vi "State wise behavior_MI.vi"(8 "error in (no error)":errorcluster, 9 "State":string, 10 "MIRecipeOpcodes":T1, 11 "VISA Refnum in":refnum<visa-resource-name>) -> (0 "error out":errorcluster, 3 "VISA Refnum out":refnum<visa-resource-name>)   [LabVIEW 2019, in "Machine Interface.lvclass"]
uses:
  Machine Interface.lvclass
  Controls/Machine Interface Config File Structure_MI.ctl
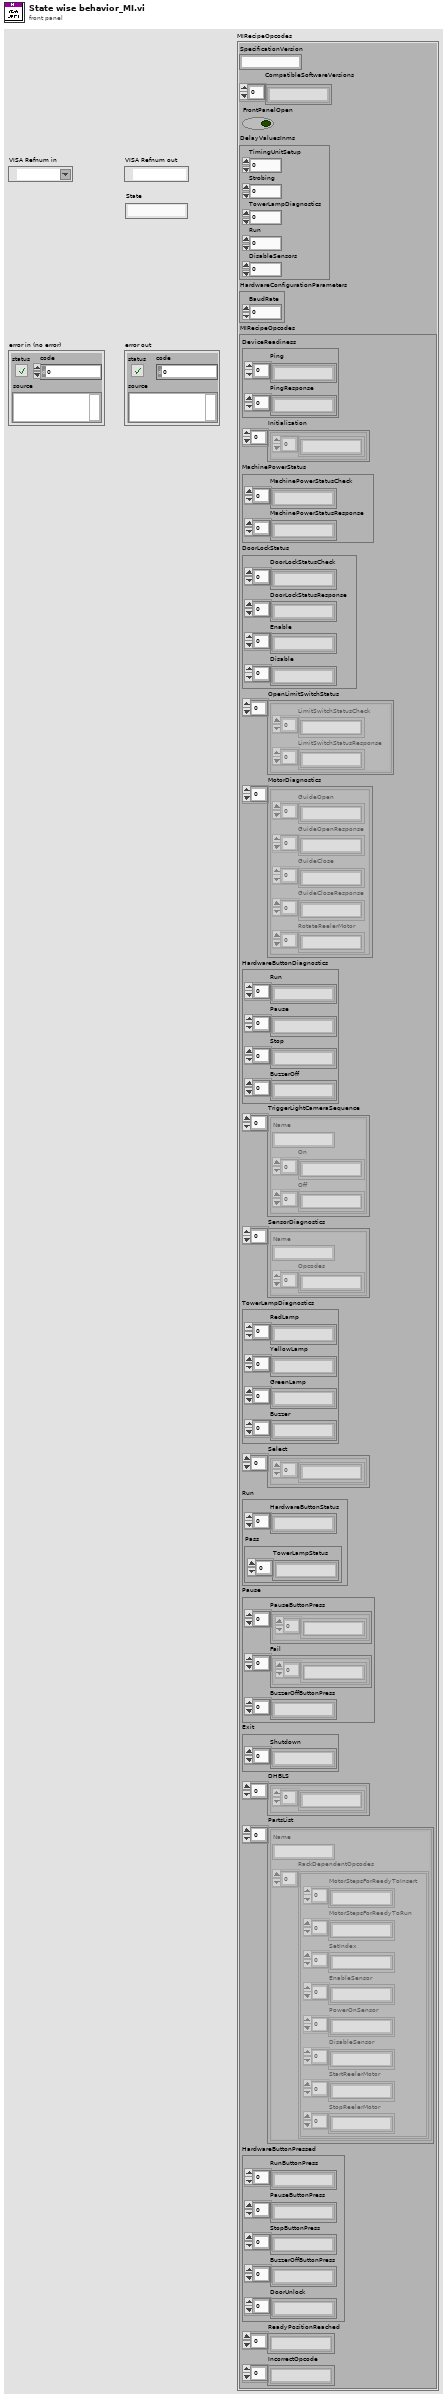
[diagram p1: front panel]
types:
  T1 = typedef "Machine Interface.lvclass/Machine Interface Config File Structure_MI.ctl" = cluster{"SpecificationVersion":string, "CompatibleSoftwareVersions":string[], "FrontPanelOpen":bool, "DelayValuesInms":cluster{"TimingUnitSetup":i32, "Strobing":i32, "TowerLampDiagnostics":i32, "Run":i32, "DisableSensors":i32}, "HardwareConfigurationParameters":cluster{"BaudRate":dbl}, "MIRecipeOpcodes":cluster{"DeviceReadiness":cluster{"Ping":string[], "PingResponse":string[]}, "Initialization":cluster{string[]}[], "MachinePowerStatus":cluster{"MachinePowerStatusCheck":string[], "MachinePowerStatusResponse":string[]}, "DoorLockStatus":cluster{"DoorLockStatusCheck":string[], "DoorLockStatusResponse":string[], "Enable":string[], "Disable":string[]}, "OpenLimitSwitchStatus":cluster{"LimitSwitchStatusCheck":string[], "LimitSwitchStatusResponse":string[]}[], "MotorDiagnostics":cluster{"GuideOpen":string[], "GuideOpenResponse":string[], "GuideClose":string[], "GuideCloseResponse":string[], "RotateReelerMotor":string[]}[], "HardwareButtonDiagnostics":cluster{"Run":string[], "Pause":string[], "Stop":string[], "BuzzerOff":string[]}, "TriggerLightCameraSequence":cluster{"Name":string, "On":string[], "Off":string[]}[], "SensorDiagnostics":cluster{"Name":string, "Opcodes":string[]}[], "TowerLampDiagnostics":cluster{"RedLamp":string[], "YellowLamp":string[], "GreenLamp":string[], "Buzzer":string[]}, "Select":cluster{string[]}[], "Run":cluster{"HardwareButtonStatus":string[], "Pass":cluster{"TowerLampStatus":string[]}}, "Pause":cluster{"PauseButtonPress":cluster{string[]}[], "Fail":cluster{string[]}[], "BuzzerOffButtonPress":string[]}, "Exit":cluster{"Shutdown":string[]}, "DHBLS":cluster{string[]}[], "PartsList":cluster{"Name":string, "RackDependentOpcodes":cluster{"MotorStepsForReadyToInsert":string[], "MotorStepsForReadyToRun":string[], "SetIndex":string[], "EnableSensor":string[], "PowerOnSensor":string[], "DisableSensor":string[], "StartReelerMotor":string[], "StopReelerMotor":string[]}[]}[], "HardwareButtonPressed":cluster{"RunButtonPress":string[], "PauseButtonPress":string[], "StopButtonPress":string[], "BuzzerOffButtonPress":string[], "DoorUnlock":string[]}, "ReadyPositionReached":string[], "IncorrectOpcode":string[]}}
  T2 = cluster{"RedLamp":string[], "YellowLamp":string[], "GreenLamp":string[], "Buzzer":string[]}
  T3 = cluster{"LimitSwitchStatusCheck":string[], "LimitSwitchStatusResponse":string[]}[]
  T4 = cluster{"LimitSwitchStatusCheck":string[], "LimitSwitchStatusResponse":string[]}
  T5 = cluster{"GuideOpen":string[], "GuideOpenResponse":string[], "GuideClose":string[], "GuideCloseResponse":string[], "RotateReelerMotor":string[]}[]
  T6 = cluster{"GuideOpen":string[], "GuideOpenResponse":string[], "GuideClose":string[], "GuideCloseResponse":string[], "RotateReelerMotor":string[]}
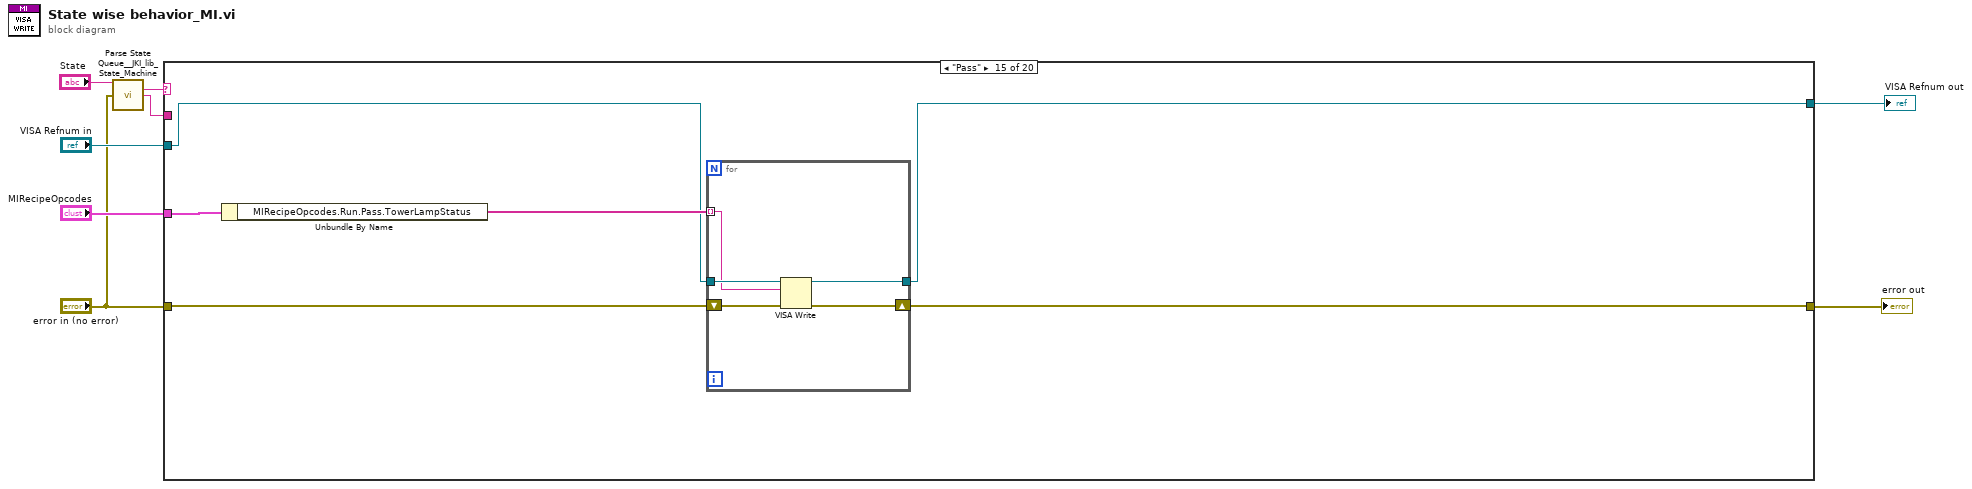
[diagram p0: block diagram]
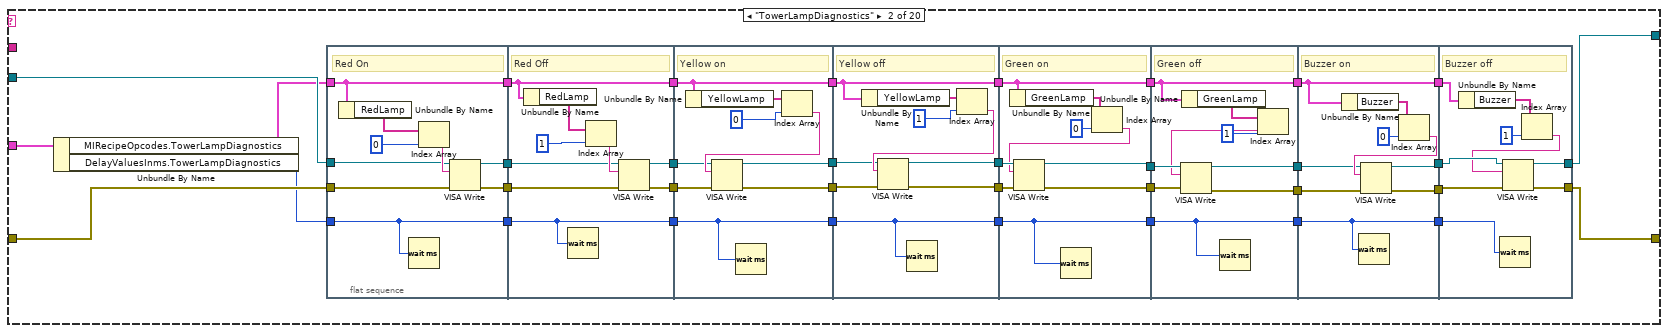
[diagram p3: hidden frame]
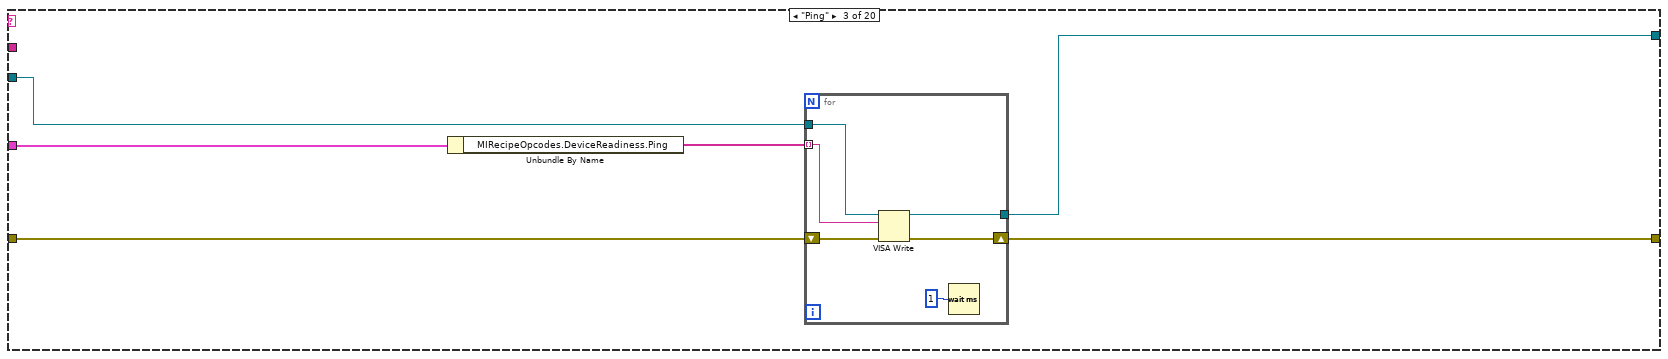
[diagram p4: hidden frame]
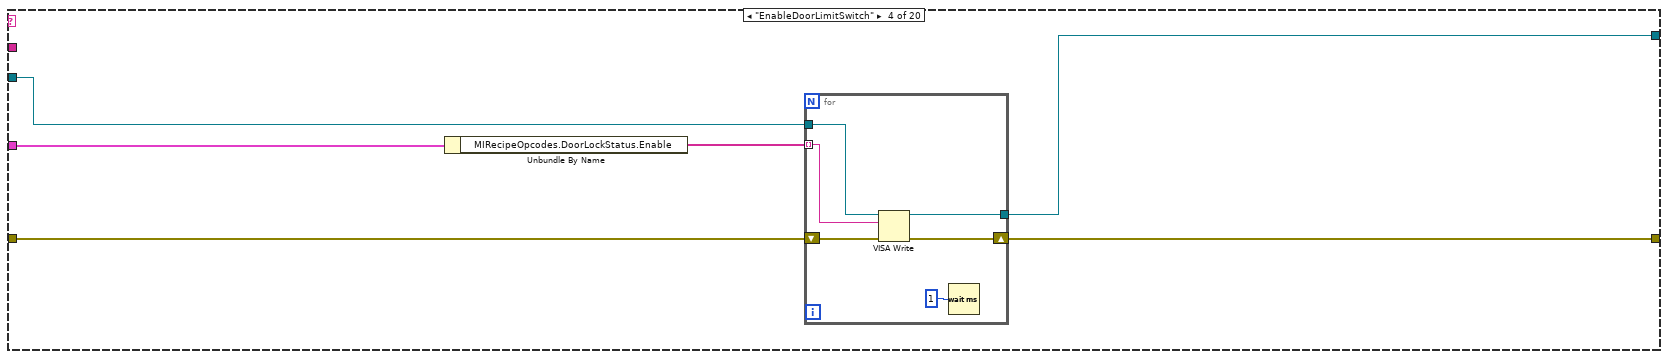
[diagram p5: hidden frame]
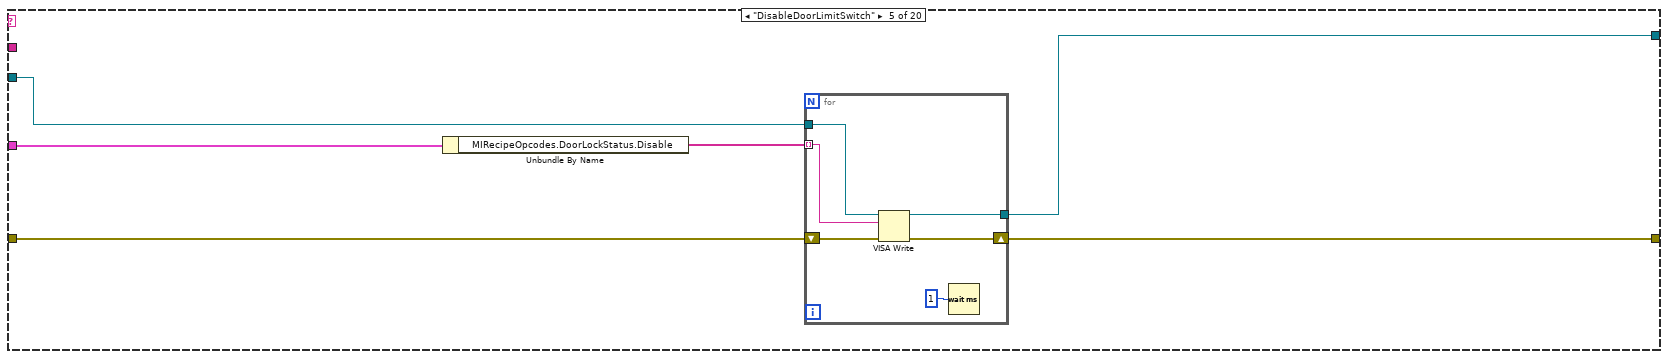
[diagram p6: hidden frame]
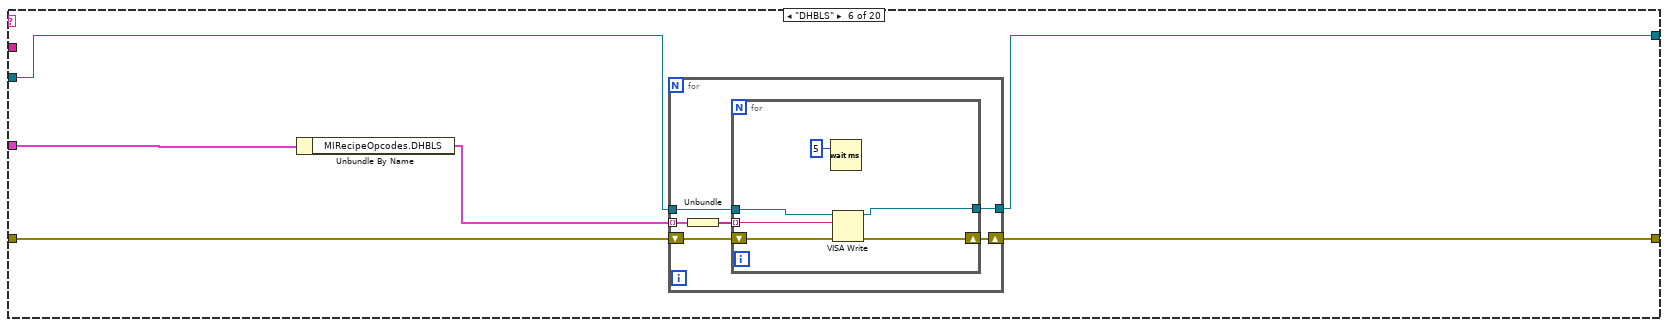
[diagram p7: hidden frame]
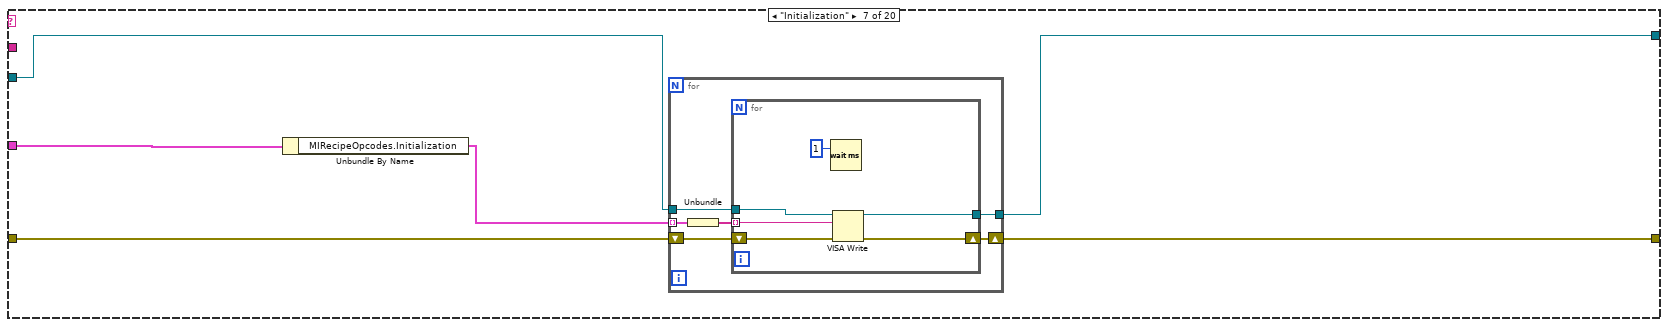
[diagram p8: hidden frame]
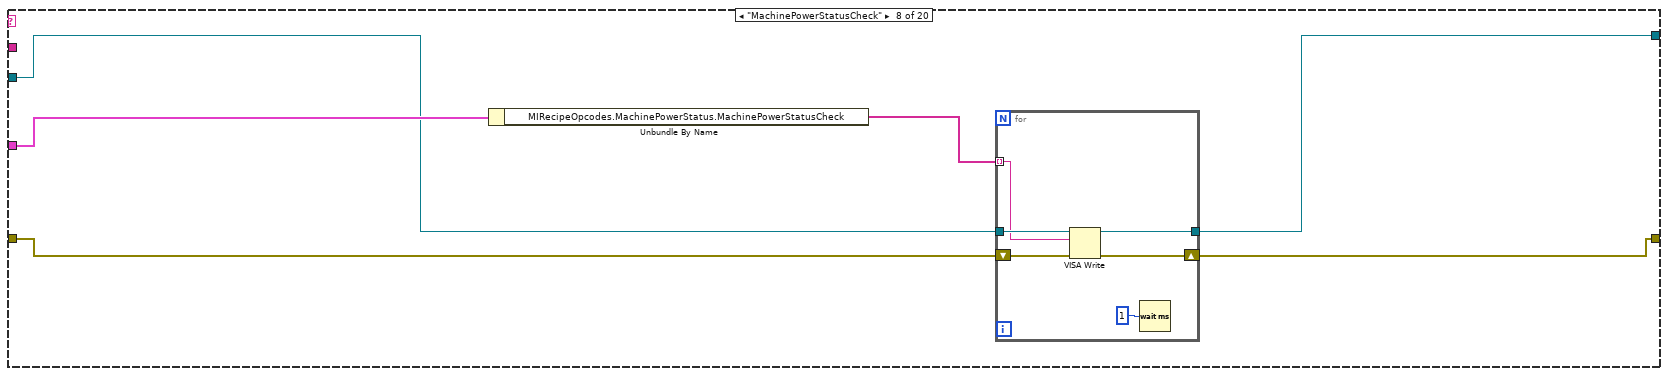
[diagram p9: hidden frame]
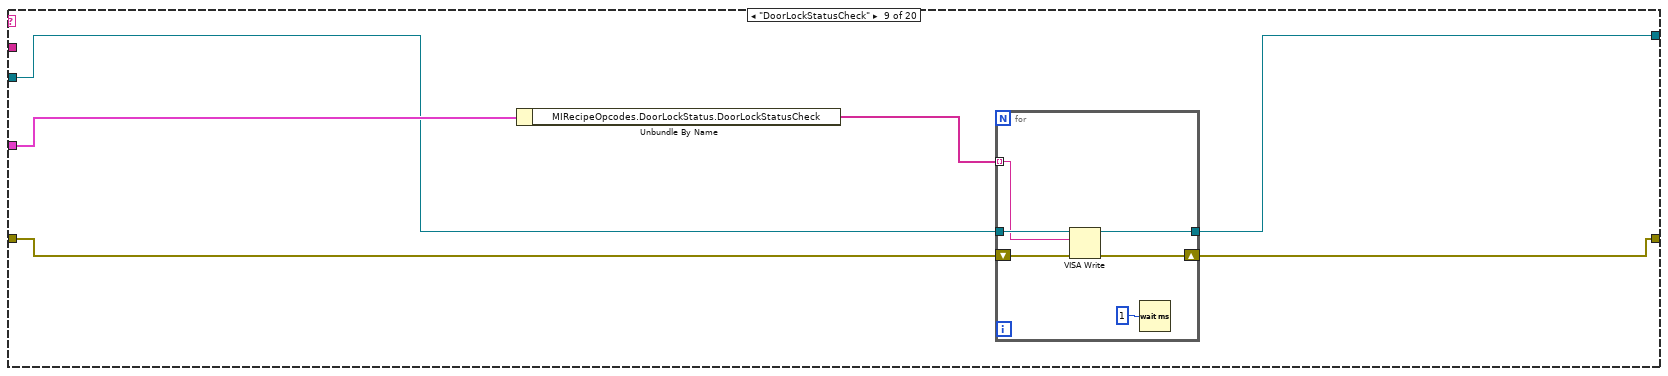
[diagram p10: hidden frame]
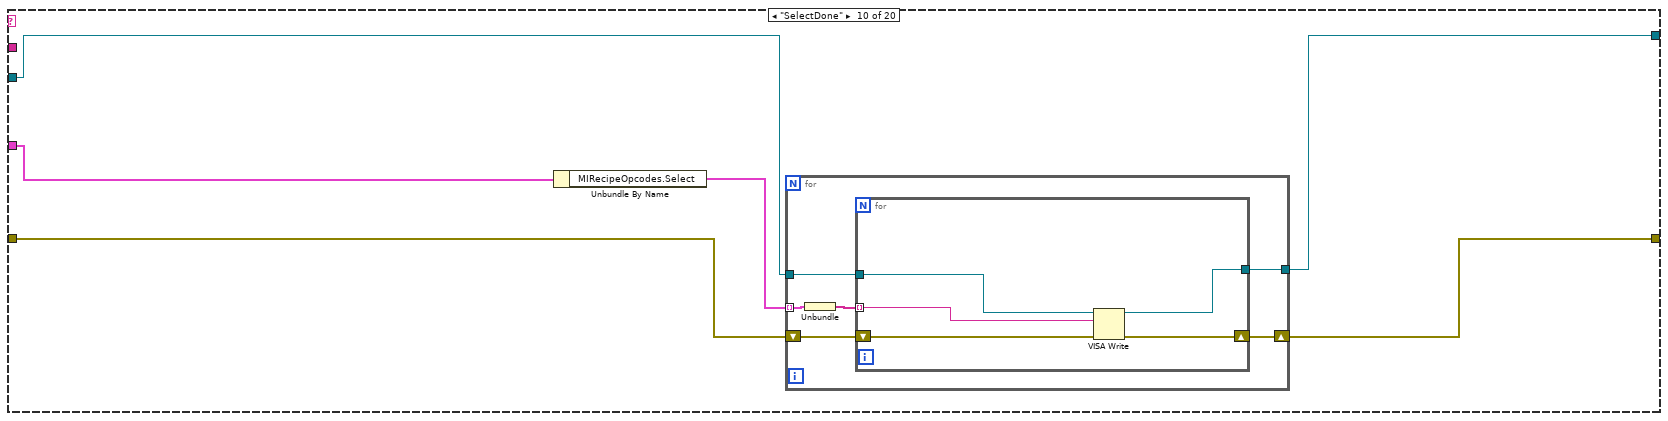
[diagram p11: hidden frame]
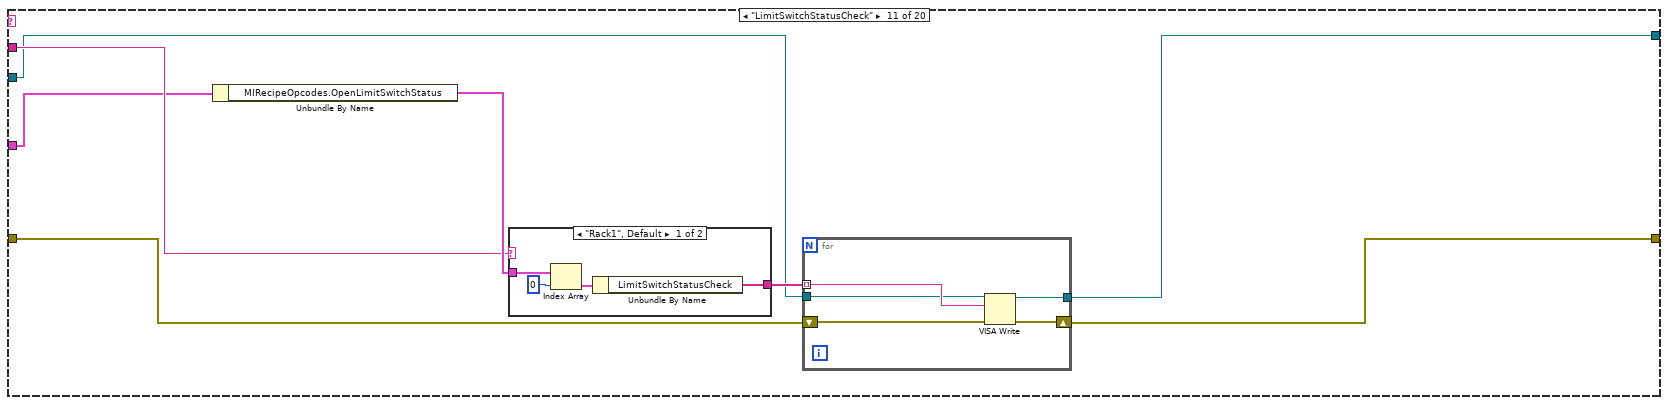
[diagram p12: hidden frame]
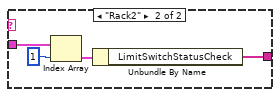
[diagram p13: hidden frame]
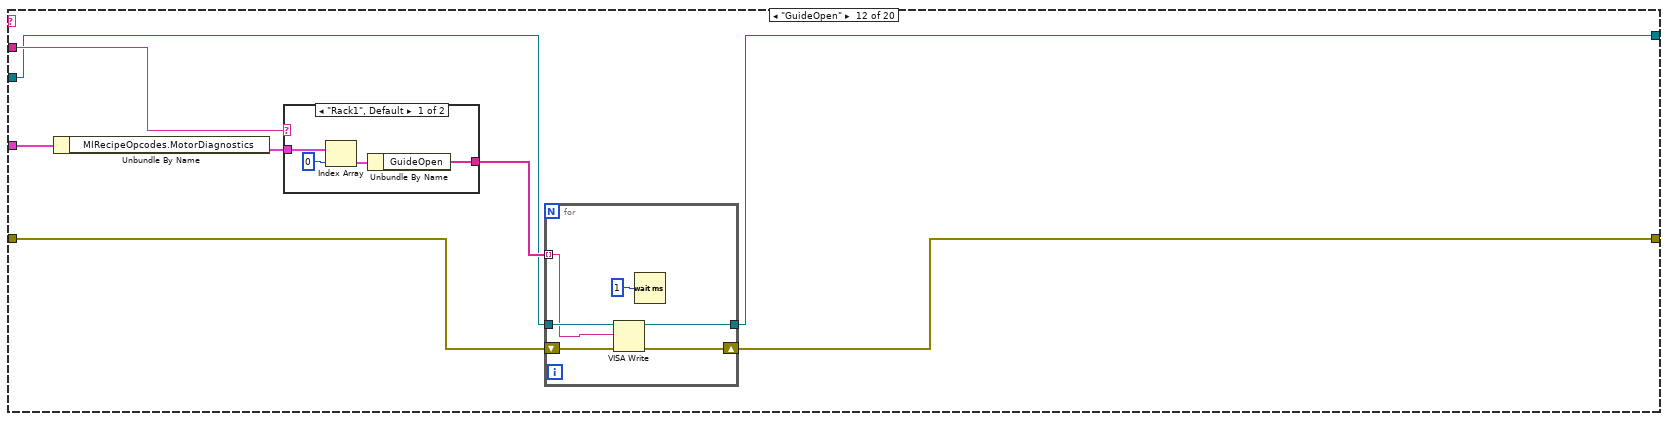
[diagram p14: hidden frame]
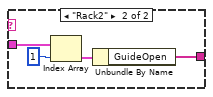
[diagram p15: hidden frame]
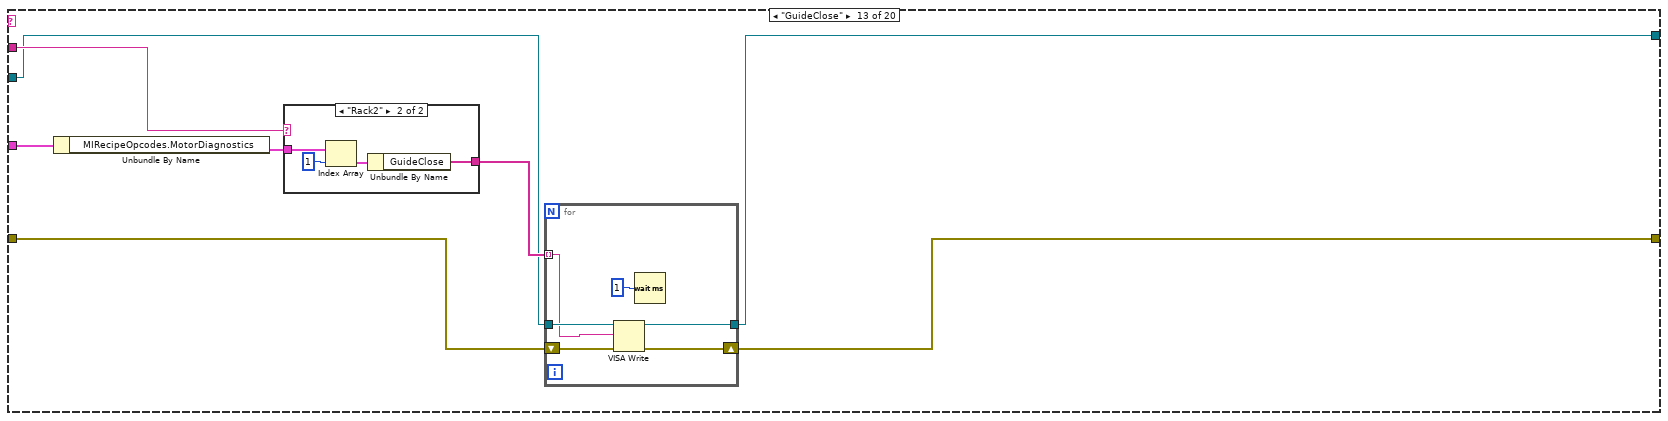
[diagram p16: hidden frame]
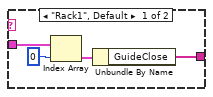
[diagram p17: hidden frame]
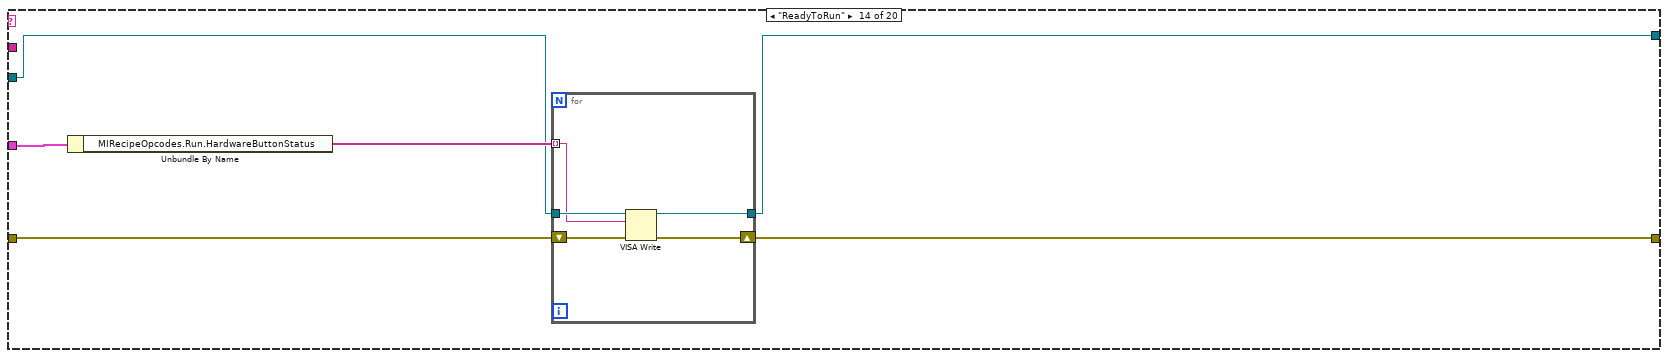
[diagram p18: hidden frame]
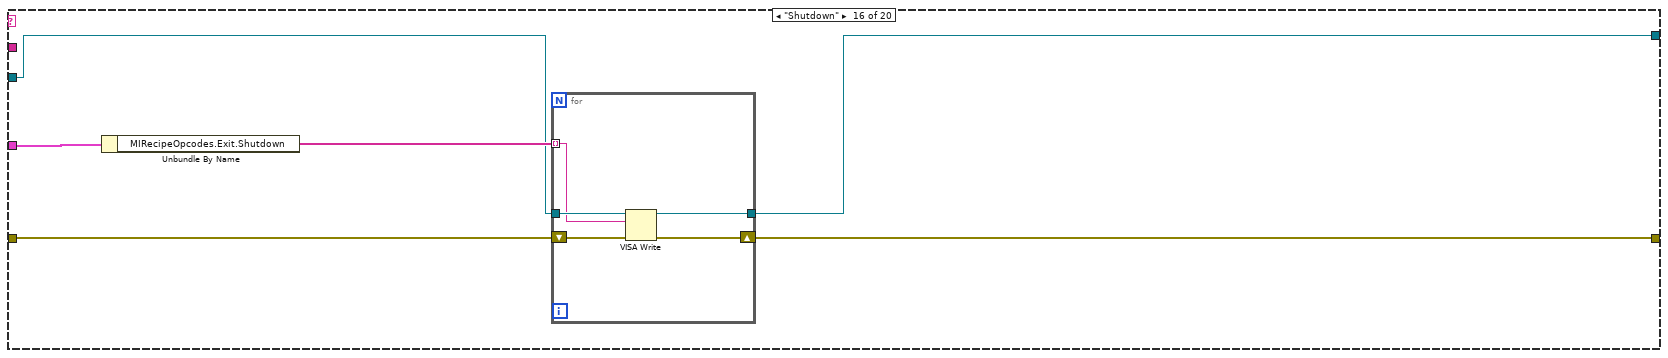
[diagram p19: hidden frame]
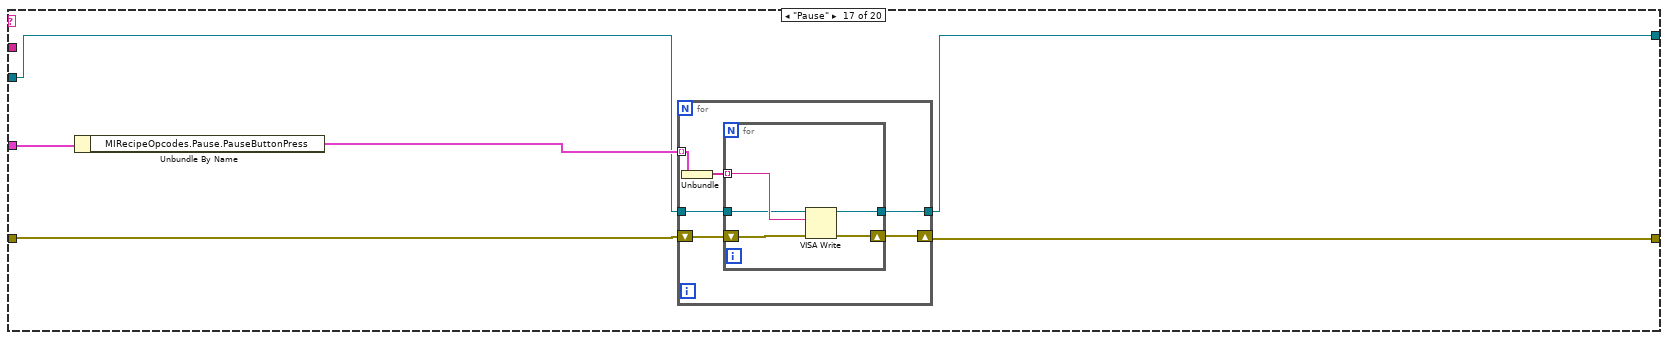
[diagram p20: hidden frame]
diagram:
  n1 = call <vilib>:"Parse State Queue__JKI_lib_State_Machine.vi"("State Queue"="State", "Error In (no error)"="error in (no error)") -> ("Current State"=w2:string, "Arguments"=w3:string)  [unwired: 11 in, 1 out]
  n2 = case shown="\"Pass\"" w2 {
    tunnel: "error in (no error)" -> [w10 w24 w121 w133 w145 w157 w175 w193 w205 w217 w234 w257 w279 w301 w312 w323 w332 w349 w368 w390]
    tunnel: [w9 w23 w118 w130 w142 w154 w172 w190 w202 w214 w231 w252 w274 w296 w307 w318 w329 w346 w363 w385] -> w8
    tunnel: [w10 w22 w120 w132 w144 w156 w174 w192 w204 w216 w233 w256 w278 w300 w311 w322 w331 w348 w367 w389] -> w1
    tunnel: "VISA Refnum in" -> [w9 w21 w119 w131 w143 w155 w173 w191 w203 w215 w232 w253 w275 w297 w308 w319 w330 w347 w364 w386]
    tunnel: "MIRecipeOpcodes" -> [_ w20 w122 w134 w146 w159 w177 w194 w206 w219 w235 w255 w277 w299 w310 w321 w334 w351 w366 w387]
    tunnel: w3 -> [_ _ _ _ _ _ _ _ _ _ w236 w258 w280 _ _ _ _ _ w369 _]
    frame Default {
    }
    frame "TowerLampDiagnostics" {
      n3 = Unbundle By Name(w20) -> ("MIRecipeOpcodes.TowerLampDiagnostics"=w19:T2, "DelayValuesInms.TowerLampDiagnostics"=w13:i32)
      n4 = flat-sequence {
        tunnel: w19 -> [w54]
        tunnel: [w54] -> w45
        tunnel: w24 -> [w51]
        tunnel: [w50] -> w44
        tunnel: w21 -> [w48]
        tunnel: [w47] -> w43
        tunnel: [w46] -> w14
        tunnel: w13 -> [w46]
        tunnel: [w58] -> w42
        tunnel: w45 -> [w58]
        tunnel: [w57] -> w41
        tunnel: w44 -> [w60]
        tunnel: w43 -> [w59]
        tunnel: [w56] -> w40
        tunnel: [w55] -> w15
        tunnel: w14 -> [w55]
        tunnel: [w69] -> w39
        tunnel: w42 -> [w69]
        tunnel: [w67] -> w38
        tunnel: w41 -> [w68]
        tunnel: w40 -> [w66]
        tunnel: [w65] -> w37
        tunnel: [w64] -> w16
        tunnel: w15 -> [w64]
        tunnel: [w78] -> w36
        tunnel: w39 -> [w78]
        tunnel: [w76] -> w35
        tunnel: w38 -> [w77]
        tunnel: w37 -> [w75]
        tunnel: [w74] -> w34
        tunnel: [w73] -> w17
        tunnel: w16 -> [w73]
        tunnel: [w90] -> w33
        tunnel: w36 -> [w90]
        tunnel: [w86] -> w32
        tunnel: w35 -> [w87]
        tunnel: w34 -> [w85]
        tunnel: [w83] -> w31
        tunnel: [w82] -> w18
        tunnel: w17 -> [w82]
        tunnel: [w99] -> w30
        tunnel: w33 -> [w99]
        tunnel: [w95] -> w29
        tunnel: w32 -> [w96]
        tunnel: w31 -> [w94]
        tunnel: [w92] -> w28
        tunnel: w18 -> [w91]
        tunnel: [w91] -> w11
        tunnel: [w108] -> w27
        tunnel: w30 -> [w108]
        tunnel: [w104] -> w26
        tunnel: w29 -> [w105]
        tunnel: w28 -> [w102]
        tunnel: [w101] -> w25
        tunnel: [w100] -> w12
        tunnel: w11 -> [w100]
        tunnel: w27 -> [w115]
        tunnel: w26 -> [w114]
        tunnel: [w113] -> w22
        tunnel: w25 -> [w112]
        tunnel: [w110] -> w23
        tunnel: w12 -> [w109]
        frame #0 {
          # "Red On"
          n5 = Unbundle By Name(w54) -> ("RedLamp"=w53:string[])
          n6 = Wait (ms)(milliseconds to wait=w46) -> ()  [unwired: 1 out]
          n7 = Index Array(array=w53, index=0) -> (element=w49:string)
          n8 = VISA Write(VISA resource name=w48, write buffer=w49, error in (no error)=w51) -> (VISA resource name out=w47:refnum<visa-resource-name>, error out=w50:errorcluster)  [unwired: 1 out]
        }
        frame #1 {
          # "Red Off"
          n9 = Unbundle By Name(w58) -> ("RedLamp"=w63:string[])
          n10 = Wait (ms)(milliseconds to wait=w55) -> ()  [unwired: 1 out]
          n11 = Index Array(array=w63, index=1) -> (element=w61:string)
          n12 = VISA Write(VISA resource name=w59, write buffer=w61, error in (no error)=w60) -> (VISA resource name out=w56:refnum<visa-resource-name>, error out=w57:errorcluster)  [unwired: 1 out]
        }
        frame #2 {
          # "Yellow on"
          n13 = Unbundle By Name(w69) -> ("YellowLamp"=w72:string[])
          n14 = Wait (ms)(milliseconds to wait=w64) -> ()  [unwired: 1 out]
          n15 = Index Array(array=w72, index=0) -> (element=w70:string)
          n16 = VISA Write(VISA resource name=w66, write buffer=w70, error in (no error)=w68) -> (VISA resource name out=w65:refnum<visa-resource-name>, error out=w67:errorcluster)  [unwired: 1 out]
        }
        frame #3 {
          # "Yellow off"
          n17 = Unbundle By Name(w78) -> ("YellowLamp"=w81:string[])
          n18 = Wait (ms)(milliseconds to wait=w73) -> ()  [unwired: 1 out]
          n19 = Index Array(array=w81, index=1) -> (element=w79:string)
          n20 = VISA Write(VISA resource name=w75, write buffer=w79, error in (no error)=w77) -> (VISA resource name out=w74:refnum<visa-resource-name>, error out=w76:errorcluster)  [unwired: 1 out]
        }
        frame #4 {
          # "Green on"
          n21 = Unbundle By Name(w90) -> ("GreenLamp"=w89:string[])
          n22 = Wait (ms)(milliseconds to wait=w82) -> ()  [unwired: 1 out]
          n23 = Index Array(array=w89, index=0) -> (element=w84:string)
          n24 = VISA Write(VISA resource name=w85, write buffer=w84, error in (no error)=w87) -> (VISA resource name out=w83:refnum<visa-resource-name>, error out=w86:errorcluster)  [unwired: 1 out]
        }
        frame #5 {
          # "Green off"
          n25 = Unbundle By Name(w99) -> ("GreenLamp"=w98:string[])
          n26 = Wait (ms)(milliseconds to wait=w91) -> ()  [unwired: 1 out]
          n27 = Index Array(array=w98, index=1) -> (element=w93:string)
          n28 = VISA Write(VISA resource name=w94, write buffer=w93, error in (no error)=w96) -> (VISA resource name out=w92:refnum<visa-resource-name>, error out=w95:errorcluster)  [unwired: 1 out]
        }
        frame #6 {
          # "Buzzer on"
          n29 = Unbundle By Name(w108) -> ("Buzzer"=w107:string[])
          n30 = Wait (ms)(milliseconds to wait=w100) -> ()  [unwired: 1 out]
          n31 = Index Array(array=w107, index=0) -> (element=w103:string)
          n32 = VISA Write(VISA resource name=w102, write buffer=w103, error in (no error)=w105) -> (VISA resource name out=w101:refnum<visa-resource-name>, error out=w104:errorcluster)  [unwired: 1 out]
        }
        frame #7 {
          # "Buzzer off"
          n33 = Unbundle By Name(w115) -> ("Buzzer"=w117:string[])
          n34 = Wait (ms)(milliseconds to wait=w109) -> ()  [unwired: 1 out]
          n35 = Index Array(array=w117, index=1) -> (element=w111:string)
          n36 = VISA Write(VISA resource name=w112, write buffer=w111, error in (no error)=w114) -> (VISA resource name out=w110:refnum<visa-resource-name>, error out=w113:errorcluster)  [unwired: 1 out]
        }
      }
    }
    frame "Ping" {
      n37 = Unbundle By Name(w122) -> ("MIRecipeOpcodes.DeviceReadiness.Ping"=w123:string[])
      n38 = for {
        tunnel: w123 -> [w128] mode=indexing
        tunnel: w119 -> [w129]
        shift-right: [w125] -> w120
        shift-left: w121 -> [w127]
        tunnel: [w124] -> w118
        n39 = VISA Write(VISA resource name=w129, write buffer=w128, error in (no error)=w127) -> (VISA resource name out=w124:refnum<visa-resource-name>, error out=w125:errorcluster)  [unwired: 1 out]
        n40 = Wait (ms)(milliseconds to wait=u32 1) -> ()  [unwired: 1 out]
      }
    }
    frame "EnableDoorLimitSwitch" {
      n41 = Unbundle By Name(w134) -> ("MIRecipeOpcodes.DoorLockStatus.Enable"=w135:string[])
      n42 = for {
        tunnel: w135 -> [w140] mode=indexing
        tunnel: w131 -> [w141]
        shift-right: [w137] -> w132
        shift-left: w133 -> [w139]
        tunnel: [w136] -> w130
        n43 = VISA Write(VISA resource name=w141, write buffer=w140, error in (no error)=w139) -> (VISA resource name out=w136:refnum<visa-resource-name>, error out=w137:errorcluster)  [unwired: 1 out]
        n44 = Wait (ms)(milliseconds to wait=u32 1) -> ()  [unwired: 1 out]
      }
    }
    frame "DisableDoorLimitSwitch" {
      n45 = Unbundle By Name(w146) -> ("MIRecipeOpcodes.DoorLockStatus.Disable"=w147:string[])
      n46 = for {
        tunnel: w147 -> [w152] mode=indexing
        tunnel: w143 -> [w153]
        shift-right: [w149] -> w144
        shift-left: w145 -> [w151]
        tunnel: [w148] -> w142
        n47 = VISA Write(VISA resource name=w153, write buffer=w152, error in (no error)=w151) -> (VISA resource name out=w148:refnum<visa-resource-name>, error out=w149:errorcluster)  [unwired: 1 out]
        n48 = Wait (ms)(milliseconds to wait=u32 1) -> ()  [unwired: 1 out]
      }
    }
    frame "DHBLS" {
      n49 = Unbundle By Name(w159) -> ("MIRecipeOpcodes.DHBLS"=w158:cluster{string[]}[])
      n50 = for {
        tunnel: w158 -> [w165] mode=indexing
        tunnel: w155 -> [w161]
        shift-right: [w162] -> w156
        shift-left: w157 -> [w163]
        tunnel: [w160] -> w154
        n51 = Unbundle(w165) -> (w164:string[])
        n52 = for {
          tunnel: w164 -> [w171] mode=indexing
          tunnel: w161 -> [w167]
          shift-right: [w168] -> w162
          shift-left: w163 -> [w169]
          tunnel: [w166] -> w160
          n53 = Wait (ms)(milliseconds to wait=u32 5) -> ()  [unwired: 1 out]
          n54 = VISA Write(VISA resource name=w167, write buffer=w171, error in (no error)=w169) -> (VISA resource name out=w166:refnum<visa-resource-name>, error out=w168:errorcluster)  [unwired: 1 out]
        }
      }
    }
    frame "Initialization" {
      n55 = Unbundle By Name(w177) -> ("MIRecipeOpcodes.Initialization"=w176:cluster{string[]}[])
      n56 = for {
        tunnel: w176 -> [w183] mode=indexing
        tunnel: w173 -> [w179]
        shift-right: [w180] -> w174
        shift-left: w175 -> [w181]
        tunnel: [w178] -> w172
        n57 = Unbundle(w183) -> (w182:string[])
        n58 = for {
          tunnel: w182 -> [w189] mode=indexing
          tunnel: w179 -> [w185]
          shift-right: [w186] -> w180
          shift-left: w181 -> [w187]
          tunnel: [w184] -> w178
          n59 = Wait (ms)(milliseconds to wait=u32 1) -> ()  [unwired: 1 out]
          n60 = VISA Write(VISA resource name=w185, write buffer=w189, error in (no error)=w187) -> (VISA resource name out=w184:refnum<visa-resource-name>, error out=w186:errorcluster)  [unwired: 1 out]
        }
      }
    }
    frame "MachinePowerStatusCheck" {
      n61 = Unbundle By Name(w194) -> ("MIRecipeOpcodes.MachinePowerStatus.MachinePowerStatusCheck"=w195:string[])
      n62 = for {
        tunnel: w195 -> [w200] mode=indexing
        tunnel: w191 -> [w201]
        shift-right: [w198] -> w192
        shift-left: w193 -> [w199]
        tunnel: [w196] -> w190
        n63 = VISA Write(VISA resource name=w201, write buffer=w200, error in (no error)=w199) -> (VISA resource name out=w196:refnum<visa-resource-name>, error out=w198:errorcluster)  [unwired: 1 out]
        n64 = Wait (ms)(milliseconds to wait=u32 1) -> ()  [unwired: 1 out]
      }
    }
    frame "DoorLockStatusCheck" {
      n65 = Unbundle By Name(w206) -> ("MIRecipeOpcodes.DoorLockStatus.DoorLockStatusCheck"=w207:string[])
      n66 = for {
        tunnel: w207 -> [w212] mode=indexing
        tunnel: w203 -> [w213]
        shift-right: [w210] -> w204
        shift-left: w205 -> [w211]
        tunnel: [w208] -> w202
        n67 = VISA Write(VISA resource name=w213, write buffer=w212, error in (no error)=w211) -> (VISA resource name out=w208:refnum<visa-resource-name>, error out=w210:errorcluster)  [unwired: 1 out]
        n68 = Wait (ms)(milliseconds to wait=u32 1) -> ()  [unwired: 1 out]
      }
    }
    frame "SelectDone" {
      n69 = Unbundle By Name(w219) -> ("MIRecipeOpcodes.Select"=w218:cluster{string[]}[])
      n70 = for {
        tunnel: w218 -> [w225] mode=indexing
        tunnel: w215 -> [w221]
        shift-right: [w222] -> w216
        shift-left: w217 -> [w223]
        tunnel: [w220] -> w214
        n71 = Unbundle(w225) -> (w224:string[])
        n72 = for {
          tunnel: w224 -> [w230] mode=indexing
          tunnel: w221 -> [w227]
          shift-right: [w228] -> w222
          shift-left: w223 -> [w229]
          tunnel: [w226] -> w220
          n73 = VISA Write(VISA resource name=w227, write buffer=w230, error in (no error)=w229) -> (VISA resource name out=w226:refnum<visa-resource-name>, error out=w228:errorcluster)  [unwired: 1 out]
        }
      }
    }
    frame "LimitSwitchStatusCheck" {
      n74 = Unbundle By Name(w235) -> ("MIRecipeOpcodes.OpenLimitSwitchStatus"=w237:T3)
      n75 = case shown="\"Rack1\", Default" w236 {
        tunnel: w237 -> [w247 w250]
        tunnel: [w244 w248] -> w238
        frame "Rack1", Default {
          n76 = Index Array(array=w247, index=0) -> (element=w245:T4)
          n77 = Unbundle By Name(w245) -> ("LimitSwitchStatusCheck"=w244:string[])
        }
        frame "Rack2" {
          n78 = Index Array(array=w250, index=1) -> (element=w249:T4)
          n79 = Unbundle By Name(w249) -> ("LimitSwitchStatusCheck"=w248:string[])
        }
      }
      n80 = for {
        tunnel: w232 -> [w240]
        tunnel: w238 -> [w241] mode=indexing
        shift-right: [w242] -> w233
        shift-left: w234 -> [w243]
        tunnel: [w239] -> w231
        n81 = VISA Write(VISA resource name=w240, write buffer=w241, error in (no error)=w243) -> (VISA resource name out=w239:refnum<visa-resource-name>, error out=w242:errorcluster)  [unwired: 1 out]
      }
    }
    frame "GuideOpen" {
      n82 = Unbundle By Name(w255) -> ("MIRecipeOpcodes.MotorDiagnostics"=w254:T5)
      n83 = case shown="\"Rack1\", Default" w258 {
        tunnel: w254 -> [w269 w271]
        tunnel: [w266 w270] -> w259
        frame "Rack1", Default {
          n84 = Index Array(array=w269, index=0) -> (element=w267:T6)
          n85 = Unbundle By Name(w267) -> ("GuideOpen"=w266:string[])
        }
        frame "Rack2" {
          n86 = Index Array(array=w271, index=1) -> (element=w272:T6)
          n87 = Unbundle By Name(w272) -> ("GuideOpen"=w270:string[])
        }
      }
      n88 = for {
        tunnel: w259 -> [w260] mode=indexing
        tunnel: w253 -> [w262]
        tunnel: [w261] -> w252
        shift-right: [w263] -> w256
        shift-left: w257 -> [w264]
        n89 = VISA Write(VISA resource name=w262, write buffer=w260, error in (no error)=w264) -> (VISA resource name out=w261:refnum<visa-resource-name>, error out=w263:errorcluster)  [unwired: 1 out]
        n90 = Wait (ms)(milliseconds to wait=u32 1) -> ()  [unwired: 1 out]
      }
    }
    frame "GuideClose" {
      n91 = Unbundle By Name(w277) -> ("MIRecipeOpcodes.MotorDiagnostics"=w276:T5)
      n92 = case shown="\"Rack2\"" w280 {
        tunnel: w276 -> [w291 w293]
        tunnel: [w288 w292] -> w281
        frame "Rack1", Default {
          n93 = Index Array(array=w291, index=0) -> (element=w289:T6)
          n94 = Unbundle By Name(w289) -> ("GuideClose"=w288:string[])
        }
        frame "Rack2" {
          n95 = Index Array(array=w293, index=1) -> (element=w294:T6)
          n96 = Unbundle By Name(w294) -> ("GuideClose"=w292:string[])
        }
      }
      n97 = for {
        tunnel: w281 -> [w282] mode=indexing
        tunnel: w275 -> [w284]
        tunnel: [w283] -> w274
        shift-right: [w285] -> w278
        shift-left: w279 -> [w286]
        n98 = VISA Write(VISA resource name=w284, write buffer=w282, error in (no error)=w286) -> (VISA resource name out=w283:refnum<visa-resource-name>, error out=w285:errorcluster)  [unwired: 1 out]
        n99 = Wait (ms)(milliseconds to wait=u32 1) -> ()  [unwired: 1 out]
      }
    }
    frame "ReadyToRun" {
      n100 = Unbundle By Name(w299) -> ("MIRecipeOpcodes.Run.HardwareButtonStatus"=w298:string[])
      n101 = for {
        tunnel: w298 -> [w305] mode=indexing
        tunnel: w297 -> [w306]
        tunnel: [w302] -> w296
        shift-right: [w303] -> w300
        shift-left: w301 -> [w304]
        n102 = VISA Write(VISA resource name=w306, write buffer=w305, error in (no error)=w304) -> (VISA resource name out=w302:refnum<visa-resource-name>, error out=w303:errorcluster)  [unwired: 1 out]
      }
    }
    frame "Pass" {
      n103 = Unbundle By Name(w310) -> ("MIRecipeOpcodes.Run.Pass.TowerLampStatus"=w309:string[])
      n104 = for {
        tunnel: w309 -> [w316] mode=indexing
        tunnel: w308 -> [w317]
        tunnel: [w313] -> w307
        shift-right: [w314] -> w311
        shift-left: w312 -> [w315]
        n105 = VISA Write(VISA resource name=w317, write buffer=w316, error in (no error)=w315) -> (VISA resource name out=w313:refnum<visa-resource-name>, error out=w314:errorcluster)  [unwired: 1 out]
      }
    }
    frame "Shutdown" {
      n106 = Unbundle By Name(w321) -> ("MIRecipeOpcodes.Exit.Shutdown"=w320:string[])
      n107 = for {
        tunnel: w320 -> [w327] mode=indexing
        tunnel: w319 -> [w328]
        shift-right: [w325] -> w322
        shift-left: w323 -> [w326]
        tunnel: [w324] -> w318
        n108 = VISA Write(VISA resource name=w328, write buffer=w327, error in (no error)=w326) -> (VISA resource name out=w324:refnum<visa-resource-name>, error out=w325:errorcluster)  [unwired: 1 out]
      }
    }
    frame "Pause" {
      n109 = Unbundle By Name(w334) -> ("MIRecipeOpcodes.Pause.PauseButtonPress"=w333:cluster{string[]}[])
      n110 = for {
        tunnel: w333 -> [w340] mode=indexing
        tunnel: w330 -> [w336]
        tunnel: [w335] -> w329
        shift-right: [w337] -> w331
        shift-left: w332 -> [w338]
        n111 = Unbundle(w340) -> (w339:string[])
        n112 = for {
          tunnel: w339 -> [w345] mode=indexing
          tunnel: w336 -> [w342]
          tunnel: [w341] -> w335
          shift-right: [w343] -> w337
          shift-left: w338 -> [w344]
          n113 = VISA Write(VISA resource name=w342, write buffer=w345, error in (no error)=w344) -> (VISA resource name out=w341:refnum<visa-resource-name>, error out=w343:errorcluster)  [unwired: 1 out]
        }
      }
    }
    frame "Fail" {
      n114 = Unbundle By Name(w351) -> ("MIRecipeOpcodes.Pause.Fail"=w350:cluster{string[]}[])
      n115 = for {
        tunnel: w350 -> [w357] mode=indexing
        tunnel: w347 -> [w353]
        tunnel: [w352] -> w346
        shift-right: [w354] -> w348
        shift-left: w349 -> [w355]
        n116 = Unbundle(w357) -> (w356:string[])
        n117 = for {
          tunnel: w356 -> [w362] mode=indexing
          tunnel: w353 -> [w359]
          tunnel: [w358] -> w352
          shift-right: [w360] -> w354
          shift-left: w355 -> [w361]
          n118 = VISA Write(VISA resource name=w359, write buffer=w362, error in (no error)=w361) -> (VISA resource name out=w358:refnum<visa-resource-name>, error out=w360:errorcluster)  [unwired: 1 out]
        }
      }
    }
    frame "RotateReelerMotor" {
      n119 = Unbundle By Name(w366) -> ("MIRecipeOpcodes.MotorDiagnostics"=w365:T5)
      n120 = case shown="\"Rack2\"" w369 {
        tunnel: w365 -> [w380 w382]
        tunnel: [w377 w381] -> w370
        frame "Rack1", Default {
          n121 = Index Array(array=w380, index=0) -> (element=w378:T6)
          n122 = Unbundle By Name(w378) -> ("RotateReelerMotor"=w377:string[])
        }
        frame "Rack2" {
          n123 = Index Array(array=w382, index=1) -> (element=w383:T6)
          n124 = Unbundle By Name(w383) -> ("RotateReelerMotor"=w381:string[])
        }
      }
      n125 = for {
        tunnel: w370 -> [w371] mode=indexing
        tunnel: w364 -> [w373]
        tunnel: [w372] -> w363
        shift-right: [w374] -> w367
        shift-left: w368 -> [w375]
        n126 = VISA Write(VISA resource name=w373, write buffer=w371, error in (no error)=w375) -> (VISA resource name out=w372:refnum<visa-resource-name>, error out=w374:errorcluster)  [unwired: 1 out]
        n127 = Wait (ms)(milliseconds to wait=u32 1) -> ()  [unwired: 1 out]
      }
    }
    frame "HardwareButtonDiagnostics" {
      w396 = 0
      w402 = ""  # Opcode
      n128 = Unbundle By Name(w387) -> ("MIRecipeOpcodes.HardwareButtonDiagnostics.Run"=w392:string[], "MIRecipeOpcodes.HardwareButtonDiagnostics.Pause"=w393:string[], "MIRecipeOpcodes.HardwareButtonDiagnostics.Stop"=w394:string[], "MIRecipeOpcodes.HardwareButtonDiagnostics.BuzzerOff"=w395:string[])
      n129 = Initialize Array(w402, 4 ("dimension size")) -> (w391:string[])
      n130 = Index Array(array=w395, index=w396) -> (element=w400:string)
      n131 = Index Array(array=w393, index=w396) -> (element=w398:string)
      n132 = Index Array(array=w392, index=w396) -> (element=w397:string)
      n133 = Index Array(array=w394, index=w396) -> (element=w399:string)
      n134 = Replace Array Subset(array=w391, new element #1=w397, new element #2=w398, new element #3=w399, new element #4=w400) -> (w388:string[])  [unwired: 4 in]
      n135 = for {
        tunnel: w386 -> [w408]
        tunnel: [w404] -> w385
        tunnel: w388 -> [w403] mode=indexing
        shift-right: [w406] -> w389
        shift-left: w390 -> [w407]
        n136 = VISA Write(VISA resource name=w408, write buffer=w403, error in (no error)=w407) -> (VISA resource name out=w404:refnum<visa-resource-name>, error out=w406:errorcluster)  [unwired: 1 out]
        n137 = Wait (ms)(milliseconds to wait=u32 1) -> ()  [unwired: 1 out]
      }
    }
  }
  "VISA Refnum out" <- w8
  "error out" <- w1
